vi "Corr2Coef Test.vi"() -> ()   [LabVIEW 2020]
panel:
  out "Corr Coef IMAQ":dbl
  out "Corr Coef U16":dbl
  out "Corr Coef IMAQ U16":dbl
  in  "B IMAQ":u16[][](array[numeric])
  in  "A":u16[][](array[numeric])
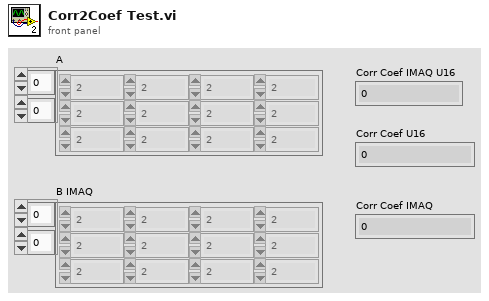
[diagram p1: front panel]
types:
  T1 = typedef "Image Type" = u32
  T2 = typedef "IMAQ Image.ctl" = refnum<image>
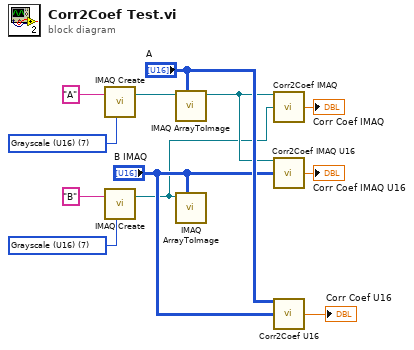
[diagram p0: block diagram]
diagram:
  w10 = T1 7 items=["Grayscale (U8)", "Grayscale (I16)", "Grayscale (SGL)", "Complex (CSG)", "RGB (U32)", "HSL (U32)", "RGB (U64)", "Grayscale (U16)"] ("Image Type")
  w11 = T1 7 items=["Grayscale (U8)", "Grayscale (I16)", "Grayscale (SGL)", "Complex (CSG)", "RGB (U32)", "HSL (U32)", "RGB (U64)", "Grayscale (U16)"] ("Image Type")
  n1 = call "IMAQ Create"("Image Name"="A", "Image Type"=w11) -> ("New Image"=w8:T2)  [unwired: 3 in, 1 out]
  n2 = call "IMAQ Create"("Image Name"="B", "Image Type"=w10) -> ("New Image"=w2:T2)  [unwired: 3 in, 1 out]
  n3 = call "IMAQ ArrayToImage"("Image Pixels (U16)"="A", "Image"=w8) -> ("Image Out"=w3:T2)  [unwired: 8 in, 1 out]
  n4 = call "IMAQ ArrayToImage"("Image Pixels (U16)"="B IMAQ", "Image"=w2) -> ()  [unwired: 8 in, 2 out]
  n5 = call "Corr2Coef IMAQ.vi"("Image A"=w3, "Image B"=w2) -> ("Corr Coef"=→"Corr Coef IMAQ":dbl)  [unwired: 12 in, 1 out]
  n6 = call "Corr2Coef IMAQ U16.vi"("Image A"=w3, "Image B"="B IMAQ") -> ("Corr Coef"=→"Corr Coef IMAQ U16":dbl)  [unwired: 12 in, 1 out]
  n7 = call "Corr2Coef U16.vi"("Image A"="A", "Image B"="B IMAQ") -> ("Corr Coef"=→"Corr Coef U16":dbl)  [unwired: 12 in, 1 out]
